vi "getCameraEventsManger.vi"(8 "error in (no error)":errorcluster, 11 "CameraController.lvclass in":refnum<class "CameraController.lvclass">) -> (0 "error out":errorcluster, 2 "Hardware:Channels.lvlib:CameraEventsManger.lvclass":refnum<class "CameraEventsManger.lvclass">, 3 "CameraController.lvclass out":refnum<class "CameraController.lvclass">)   [LabVIEW 2009, in "Hardware.lvlib" / "Channels.lvlib" / "CameraController.lvclass"]
uses:
  CameraController.lvclass
  CameraEventsManager/CameraEventsManger.lvclass
  CameraController.lvclass/CameraController.ctl
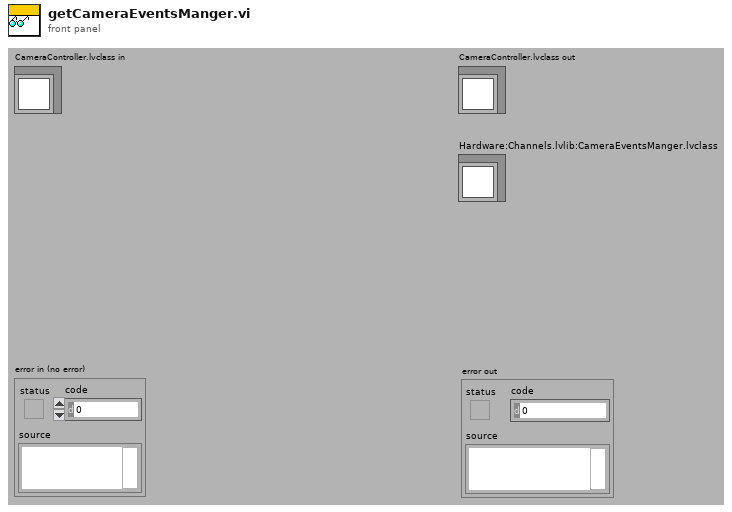
[diagram p1: front panel]
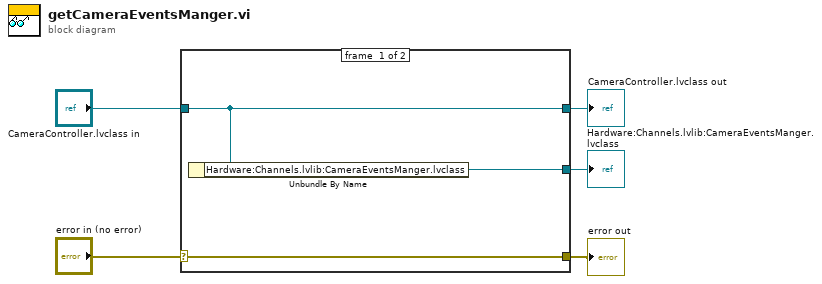
[diagram p0: block diagram]
diagram:
  n1 = case shown="No Error" "error in (no error)" {
    selector: "error in (no error)" -> [w8 w9]
    tunnel: [w8 w9] -> w1
    tunnel: [w7 w10] -> w3
    tunnel: "CameraController.lvclass in" -> [w7 w10]
    tunnel: [w6 _] -> w2
    frame #0 {
      n2 = Unbundle By Name(w7) -> ("Hardware:Channels.lvlib:CameraEventsManger.lvclass"=w6:refnum<class "CameraEventsManger.lvclass">)
    }
    frame #1 {
    }
  }
  "CameraController.lvclass out" <- w3
  "Hardware:Channels.lvlib:CameraEventsManger.lvclass" <- w2
  "error out" <- w1
